vi "experiment control.vi"() -> ()   [LabVIEW 2012] (continued)
                n2481 = Concatenate Strings("ST" ("string"), w5561, "MS" ("string")) -> (w5558:string)
                n2482 = VISA Write(VISA resource name=w5564, write buffer=w5558, error in (no error)=w5565) -> (VISA resource name out=w5563:refnum<visa-resource-name>, error out=w5566:errorcluster)  [unwired: 1 out]
                n2483 = Bundle By Name(cluster=w5568, "GPIB Port"=w5563) -> (w5567:T27)
                n2484 = local write "HP8341B"(w5567) -> ()
              }
            }
          }
          frame "Microwave: Set Sweep" {
            # "Use this as a template for any command that you might want to profile."
            n2485 = local read "HP8341B"() -> (w5573:T27)
            n2486 = Unbundle By Name(w5573) -> ("detected"=w5570:bool, "Chirp"=w5571:bool)
            n2487 = And(x=w5570, y=w5571) -> (x .and. y?=w5572:bool)
            n2488 = case shown="True" w5572 {
              tunnel: w5573 -> [_ w5594]
              tunnel: [w5577 w5592] -> w5574
              tunnel: w5575 -> [w5577 w5591]
              frame False {
              }
              frame True {
                n2489 = Unbundle By Name(w5594) -> ("GPIB Port"=w5590:refnum<visa-resource-name>, "Set frequency"=w5588:dbl, "stop frequency"=w5584:dbl)
                n2490 = Number To Fractional String(number=w5588) -> (F-format string=w5587:string)  [unwired: 3 in]
                n2491 = Number To Fractional String(number=w5584) -> (F-format string=w5581:string)  [unwired: 3 in]
                n2492 = Concatenate Strings("FA" ("string"), w5587, "MZ" ("string"), "FB" ("string"), w5581, "MZ" ("string"), "S1" ("string"), "T3" ("string")) -> (w5585:string)
                n2493 = VISA Write(VISA resource name=w5590, write buffer=w5585, error in (no error)=w5591) -> (VISA resource name out=w5589:refnum<visa-resource-name>, error out=w5592:errorcluster)  [unwired: 1 out]
                n2494 = Bundle By Name(cluster=w5594, "GPIB Port"=w5589) -> (w5593:T27)
                n2495 = local write "HP8341B"(w5593) -> ()
              }
            }
          }
        }
      }
      frame #2 {
        n2496 = Unbundle By Name(w5599) -> ("Command Names"=w5603:string[])
        n2497 = Tick Count (ms)() -> (millisecond timer value=w5604:u32)
        n2498 = Search 1D Array(1D array=w5603, element=w5600) -> (index of element=w5596:i32)  [unwired: 1 in]
        n2499 = Subtract(x=w5604, y=w5598) -> (x-y=w5602:u32)
        n2500 = local read "debug timing"() -> (w5597:cluster{"command":string, "time":dbl}[])
        n2501 = Bundle("Current State"=w5600, w5602) -> (w5595:cluster{"Current State":string, u32})  [unwired: 1 in]
        n2502 = Greater Or Equal To 0?(x=w5596) -> (x >= 0?=w5601:bool)
        n2503 = case shown="False" w5601 {
          tunnel: w5597 -> [_ w5608]
          tunnel: w5596 -> [_ w5607]
          tunnel: w5595 -> [_ w5605]
          frame False {
          }
          frame True {
            n2504 = Replace Array Subset(array=w5608, new element=w5605, index=w5607) -> (→"debug timing":cluster{"command":string, "time":dbl}[])
          }
        }
      }
    }
  }
  n2505 = disable-structure shown="Enabled" {
    disable-tunnel: w1 -> [w5609 _]
    frame Enabled {
      n2506 = while "User Interface Loop" {
        tunnel: w5609 -> [w5613]
        stop <- w5610 stop-if-true
        n2507 = event shown="[13] \"save\": Value Change" {
          selector: _ -> [_ _ _ _ _ _ _ _ _ _ _ _ _ _ _ _ _ _ _ _ _ _ _ _ _ _ _ _ _ _ _ _ _ _ _ _ _ _ _ _ _ _ _ _ _ _ _ _ _ _ _ _ _ _ _ _ _ _ _ _ _ _ _]
          dyn-events: _ -> [_ _ _ _ _ _ _ _ _ _ _ _ _ _ _ _ _ _ _ _ _ _ _ _ _ _ _ _ _ _ _ _ _ _ _ _ _ _ _ _ _ _ _ _ _ _ _ _ _ _ _ _ _ _ _ _ _ _ _ _ _ _ _]
          timeout: 1000 -> [_ _ _ _ _ _ _ _ _ _ _ _ _ _ _ _ _ _ _ _ _ _ _ _ _ _ _ _ _ _ _ _ _ _ _ _ _ _ _ _ _ _ _ _ _ _ _ _ _ _ _ _ _ _ _ _ _ _ _ _ _ _ _]
          tunnel: w5613 -> [w5617 w5631 w5660 w5670 w5672 w5794 w5803 w5805 w5809 w5812 w5815 w5818 w5821 w5824 w5830 w5833 w5836 w5839 w5842 w5848 w5854 w5861 w5864 w5893 w5911 w5933 w5940 w5970 w5973 w5976 w5979 w5982 w5986 w5993 w6004 w6010 w6013 w6019 w6022 w6025 w6028 w6031 w6037 w6040 w6043 w6046 w6049 w6052 w6055 w6058 w6061 w6070 w6079 w6088 w6097 w6102 w6108 w6113 w6116 w6119 w6122 w6123 w6152]
          tunnel: [w5617 w5631 w5660 w5670 w5672 w5794 w5802 w5804 w5808 w5811 w5814 w5817 w5820 w5823 w5829 w5832 w5835 w5838 w5841 w5848 w5853 w5860 w5863 w5893 w5910 w5933 w5940 w5969 w5972 w5975 w5978 w5981 w5985 w5992 w6003 w6009 w6012 w6018 w6021 w6024 w6027 w6030 w6036 w6039 w6042 w6045 w6048 w6051 w6054 w6057 w6060 w6069 w6078 w6087 w6096 w6101 w6107 w6112 w6115 w6118 w6121 w6123 w6151] -> w5611
          event Timeout {
            n2508 = event-data() -> ()  [unwired: 1 in, 2 out]
            n2509 = Get Date/Time String(want seconds? (F)=TRUE) -> (date string=w5623:string, time string=w5624:string)  [unwired: 2 in]
            n2510 = Get Queue Status(queue=w5617, return elements? (F)=TRUE) -> (error out=w5616:errorcluster, elements=w5621:string[])  [unwired: 1 in, 6 out]
            n2511 = local write "Time"(w5624) -> ()
            n2512 = local write "Date"(w5623) -> ()
            n2513 = Search 1D Array(1D array=w5621, element="Idle") -> (index of element=w5619:i32)  [unwired: 1 in]
            n2514 = Less Than 0?(x=w5619) -> (x < 0?=w5618:bool)
            n2515 = case shown="True" w5618 {
              tunnel: w5617 -> [_ w5630]
              tunnel: w5616 -> [w5626 w5628]
              tunnel: [w5626 w5627] -> w5615
              frame False {
              }
              frame True {
                n2516 = Enqueue Element(queue=w5630, element="Idle", error in (no error)=w5628) -> (error out=w5627:errorcluster)  [unwired: 1 in, 2 out]
              }
            }
            n2517 = call <vilib>:"Clear Errors.vi"("error in (no error)"=w5615) -> ()  [unwired: 6 in, 1 out]
          }
          event Menu Selection (User) {
            n2518 = event-data() -> ("ItemTag"=w5632:string)  [unwired: 1 in]
            n2519 = case shown="\"Save\"" w5632 {
              tunnel: w5631 -> [_ w5634 w5636 w5638 w5645 w5654 w5656]
              frame "", Default {
              }
              frame "Save" {
                n2520 = Enqueue Element At Opposite End(queue=w5634, element="uBinary: Save >> Prompt") -> ()  [unwired: 2 in, 3 out]
              }
              frame "Load" {
                n2521 = Enqueue Element At Opposite End(queue=w5636, element="uBinary: Load") -> ()  [unwired: 2 in, 3 out]
              }
              frame "Abort" {
                n2522 = Enqueue Element At Opposite End(queue=w5638, element="Abort") -> ()  [unwired: 2 in, 3 out]
              }
              frame "Test" {
                w5640 = "Test" ("item tag")
                n2523 = Current VI's Menubar() -> (w5641:refnum<k9>)
                n2524 = Get Menu Item Info(7:w5640, 11:w5641) -> (0:w5642:errorcluster, 3:w5644:refnum<k9>, 4:w5643:bool)  [unwired: 1 in, 4 out]
                n2525 = Not(x=w5643) -> (.not. x?=w5639:bool)
                n2526 = Set Menu Item Info(6:w5639, 7:w5640, 8:w5642, 11:w5644) -> ()  [unwired: 3 in, 2 out]
                n2527 = case shown="True" w5639 {
                  tunnel: w5645 -> [_ w5647]
                  tunnel: w5640 -> [_ w5646]
                  frame False {
                  }
                  frame True {
                    n2528 = Enqueue Element At Opposite End(queue=w5647, element=w5646) -> ()  [unwired: 2 in, 3 out]
                  }
                }
              }
              frame "Pause" {
                w5649 = "Pause" ("item tag")
                n2529 = Current VI's Menubar() -> (w5650:refnum<k9>)
                n2530 = Get Menu Item Info(7:w5649, 11:w5650) -> (0:w5651:errorcluster, 3:w5653:refnum<k9>, 4:w5652:bool)  [unwired: 1 in, 4 out]
                n2531 = Not(x=w5652) -> (.not. x?=w5648:bool)
                n2532 = Set Menu Item Info(6:w5648, 7:w5649, 8:w5651, 11:w5653) -> ()  [unwired: 3 in, 2 out]
                n2533 = Enqueue Element At Opposite End(queue=w5654, element=w5649) -> ()  [unwired: 2 in, 3 out]
              }
              frame "Quit" {
                n2534 = Enqueue Element At Opposite End(queue=w5656, element="Macro: Exit") -> ()  [unwired: 2 in, 3 out]
              }
            }
          }
          event "Help Function Names": Double Click {
            n2535 = event-data() -> ("Row"=w5659:i32)  [unwired: 1 in]
            n2536 = property on="Help Function Names" class="LstBox (strict)"() -> ("Item Names"=w5658:string[])  [unwired: 2 in, 2 out]
            n2537 = Index Array(array=w5658, index=w5659) -> (element=w5657:string)
            n2538 = local write "stdin"(w5657) -> ()
          }
          event Shortcut Menu Activation? {
            n2539 = event-data() -> ("MenuRef"=w5663:refnum<k9>, "SubObj"=w5662:refnum<vi>)  [unwired: 1 in]
            n2540 = property class="Ctl"(reference=w5662) -> (error out=w5665:errorcluster, "Label.Text"=w5668:string)  [unwired: 1 in, 1 out]
            n2541 = Concatenate Strings("Load ", w5668, " from uBinary" ("string")) -> (w5666:string)
            n2542 = Insert Menu Items(4:w5666, 6:w5665, 8:w5666, 9:w5663) -> (0:w5664:errorcluster)  [unwired: 2 in, 2 out]
            n2543 = call <vilib>:"Clear Errors.vi"("error in (no error)"=w5664) -> ()  [unwired: 6 in, 1 out]
            n2544 = event-data("Discard?"=FALSE) -> ()  [unwired: 1 in, 1 out]
          }
          event Shortcut Menu Selection (User) {
            n2545 = event-data() -> ("ItemTag"=w5671:string)  [unwired: 1 in]
            n2546 = xnode "Match Regular Expression"("input string"=w5671, "regular expression"="Load (.+) from uBinary") -> ("offset past match"=w5675:i32, "submatch 1"=w5673:string)  [unwired: 4 in, 4 out]
            n2547 = Greater Or Equal To 0?(x=w5675) -> (x >= 0?=w5674:bool)
            n2548 = case shown="True" w5674 {
              tunnel: w5672 -> [_ w5680]
              tunnel: w5673 -> [_ w5678]
              frame False {
              }
              frame True {
                n2549 = Concatenate Strings("uBinary: Load >> " ("string"), w5678) -> (w5679:string)
                n2550 = Enqueue Element At Opposite End(queue=w5680, element=w5679) -> ()  [unwired: 2 in, 3 out]
              }
            }
          }
          event "stdin": Key Down {
            n2551 = event-data() -> ("ScanCode"=w5795:i16)  [unwired: 1 in]
            n2552 = case shown="28" w5795 {
              tunnel: w5794 -> [_ w5796]
              frame 0, Default {
              }
              frame 28 {
                # "User Presses Enter"
                n2553 = stacked-sequence {
                  tunnel: [_ w5799 _] -> w5797
                  frame #0 {
                    n2554 = property on="stdin" class="Str"("Text.Selection"=T116 {"Selection Start"=0, "Selection End"=4294967295}) -> ()  [unwired: 2 in, 2 out]
                  }
                  frame #1 {
                    n2555 = local read "stdin"() -> (w5799:string)
                  }
                  frame #2 {
                    n2556 = property on="stdin" class="Str"("Key Focus"=TRUE) -> ()  [unwired: 2 in, 2 out]
                  }
                }
                n2557 = Enqueue Element At Opposite End(queue=w5796, element=w5797) -> ()  [unwired: 2 in, 3 out]
              }
            }
          }
          event "State Hierarchy", "Machine State": Value Change {
            n2558 = event-data() -> ()  [unwired: 1 in, 5 out]
            n2559 = Enqueue Element(queue=w5803, element="Switch: Update Hierarchy") -> (queue out=w5802:refnum<queue>)  [unwired: 2 in, 2 out]
          }
          event "stop": Value Change {
            # "Exit Button Value Change (pressed) Event\n(this executes Macro: Exit to terminate the VI)"
            n2560 = event-data() -> ()  [unwired: 1 in, 5 out]
            n2561 = Enqueue Element At Opposite End(queue=w5805, element="Macro: Exit") -> (queue out=w5804:refnum<queue>)  [unwired: 2 in, 2 out]
          }
          event "Machine State.Brot": Value Change {
            n2562 = event-data() -> ()  [unwired: 1 in, 5 out]
            n2563 = Enqueue Element At Opposite End(queue=w5809, element="Switch: Set >> Brot" ("State(s) in Front (\"\")")) -> (queue out=w5808:refnum<queue>)  [unwired: 2 in, 2 out]
          }
          event "Machine State.Doublet": Value Change {
            n2564 = event-data() -> ()  [unwired: 1 in, 5 out]
            n2565 = Enqueue Element At Opposite End(queue=w5812, element="Switch: Set >> Doublet" ("State(s) in Front (\"\")")) -> (queue out=w5811:refnum<queue>)  [unwired: 2 in, 2 out]
          }
          event "Machine State.Rotation": Value Change {
            n2566 = event-data() -> ()  [unwired: 1 in, 5 out]
            n2567 = Enqueue Element At Opposite End(queue=w5815, element="Switch: Set >> Rotation" ("State(s) in Front (\"\")")) -> (queue out=w5814:refnum<queue>)  [unwired: 2 in, 2 out]
          }
          event "Machine State.Depletion phase": Value Change {
            n2568 = event-data() -> ()  [unwired: 1 in, 5 out]
            n2569 = Enqueue Element At Opposite End(queue=w5818, element="Switch: Set >> Depletion phase" ("State(s) in Front (\"\")")) -> (queue out=w5817:refnum<queue>)  [unwired: 2 in, 2 out]
          }
          event "Machine State.Depletion pol": Value Change {
            n2570 = event-data() -> ()  [unwired: 1 in, 5 out]
            n2571 = Enqueue Element At Opposite End(queue=w5821, element="Switch: Set >> Readout" ("State(s) in Front (\"\")")) -> (queue out=w5820:refnum<queue>)  [unwired: 2 in, 2 out]
          }
          event "save": Value Change {
            n2572 = event-data() -> ()  [unwired: 1 in, 5 out]
            n2573 = Enqueue Element At Opposite End(queue=w5824, element="uBinary: Save >> Prompt" ("State(s) in Front (\"\")")) -> (queue out=w5823:refnum<queue>)  [unwired: 2 in, 2 out]
          }
          event "TiSapph.setpoint": Value Change {
            n2574 = event-data() -> ()  [unwired: 1 in, 5 out]
            n2575 = local read "TiSapph"() -> (w5825:T18)
            n2576 = Unbundle By Name(w5825) -> ("setpoint"=w5827:dbl)
            n2577 = Bundle By Name(cluster=w5825, "scan start"=w5827) -> (w5826:T18)
            n2578 = Enqueue Element At Opposite End(queue=w5830, element="Laser: Start Scan >> TiSapph" ("State(s) in Front (\"\")")) -> (queue out=w5829:refnum<queue>)  [unwired: 2 in, 2 out]
            n2579 = local write "TiSapph"(w5826) -> ()
          }
          event "load": Value Change {
            n2580 = event-data() -> ()  [unwired: 1 in, 5 out]
            n2581 = Enqueue Element At Opposite End(queue=w5833, element="uBinary: Load" ("State(s) in Front (\"\")")) -> (queue out=w5832:refnum<queue>)  [unwired: 2 in, 2 out]
          }
          event "Trap DDS.channels": Value Change {
            n2582 = event-data() -> ()  [unwired: 1 in, 5 out]
            n2583 = Enqueue Element At Opposite End(queue=w5836, element="Trap DDS: Upload" ("State(s) in Front (\"\")")) -> (queue out=w5835:refnum<queue>)  [unwired: 2 in, 2 out]
          }
          event "DIO64 Override": Value Change {
            n2584 = event-data() -> ()  [unwired: 1 in, 5 out]
            n2585 = Enqueue Element At Opposite End(queue=w5839, element="DIO64: Override" ("State(s) in Front (\"\")")) -> (queue out=w5838:refnum<queue>)  [unwired: 2 in, 2 out]
          }
          event "DIO64 Tasks": Value Change {
            n2586 = event-data() -> ()  [unwired: 1 in, 5 out]
            n2587 = Enqueue Element At Opposite End(queue=w5842, element="UI: DIO64 Update Control" ("State(s) in Front (\"\")")) -> (queue out=w5841:refnum<queue>)  [unwired: 2 in, 2 out]
          }
          event "Trap DDS.ioupdate": Value Change {
            n2588 = event-data() -> ()  [unwired: 1 in, 5 out]
            n2589 = local read "Trap DDS"() -> (w5845:T26)
            n2590 = Unbundle By Name(w5845) -> ("usb 1"=w5843:refnum<visa-resource-name>, "usb 2"=w5844:refnum<visa-resource-name>)
            n2591 = Bundle By Name(cluster=w5845, "ioupdate"=FALSE) -> (w5847:T26)
            n2592 = call "DDS9959 IO Update.vi"("VISA resource name"=w5843) -> ()  [unwired: 5 in, 2 out]
            n2593 = call "DDS9959 IO Update.vi"("VISA resource name"=w5844) -> ()  [unwired: 5 in, 2 out]
            n2594 = local write "Trap DDS"(w5847) -> ()
          }
          event "Abort": Value Change {
            n2595 = event-data() -> ()  [unwired: 1 in, 5 out]
            n2596 = Enqueue Element At Opposite End(queue=w5854, element="Abort") -> (queue out=w5853:refnum<queue>)  [unwired: 2 in, 2 out]
            n2597 = call <vilib>:"Create Rendezvous.vi"("return existing (F)"=TRUE, "name (unnamed)"="sync") -> ("error out"=w5852:errorcluster, "rendezvous"=w5850:T56)  [unwired: 3 in, 1 out]
            n2598 = case shown="No Error" w5852 {
              tunnel: w5850 -> [w5857 _]
              tunnel: w5852 -> [w5856 w5858]
              frame No Error {
                n2599 = call <vilib>:"Wait at Rendezvous.vi"("error in (no error)"=w5856, "rendezvous"=w5857) -> ()  [unwired: 3 in, 3 out]
              }
              frame Error {
                n2600 = call <vilib>:"Clear Errors.vi"("error in (no error)"=w5858) -> ()  [unwired: 6 in, 1 out]
              }
            }
          }
          event "Test": Value Change {
            n2601 = event-data() -> ()  [unwired: 1 in, 5 out]
            n2602 = Enqueue Element At Opposite End(queue=w5861, element="Test") -> (queue out=w5860:refnum<queue>)  [unwired: 2 in, 2 out]
          }
          event "Measure": Value Change {
            n2603 = event-data() -> ()  [unwired: 1 in, 5 out]
            n2604 = local read "Measure Commands"() -> (w5866:string)
            n2605 = while {
              shift-right: [w5875] -> _
              shift-left: w5866 -> [w5877]
              tunnel: [w5874] -> w5862 mode=indexing
              stop <- w5872 stop-if-true
              n2606 = Match Pattern(string=w5877, regular expression="[\\n\\r]+") -> (before substring=w5874:string, after substring=w5875:string, offset past match=w5873:i32)  [unwired: 1 in, 1 out]
              n2607 = Less Than 0?(x=w5873) -> (x < 0?=w5872:bool)
            }
            n2608 = for {
              tunnel: [w5871] -> w5863
              tunnel: w5864 -> [w5870]
              shift-right: [w5868] -> w5865
              shift-left: _ -> [w5869]
              tunnel: w5862 -> [w5867] mode=indexing
              n2609 = Enqueue Element(queue=w5870, element=w5867, error in (no error)=w5869) -> (queue out=w5871:refnum<queue>, error out=w5868:errorcluster)  [unwired: 1 in, 1 out]
            }
            n2610 = call <vilib>:"Clear Errors.vi"("error in (no error)"=w5865) -> ()  [unwired: 6 in, 1 out]
          }
          event "DIO64 Tasks": Mouse Down {
            n2611 = event-data() -> ("Button"=w5878:u16, "Coords.Vertical"=w5879:i32)  [unwired: 1 in]
            n2612 = property on="DIO64 Tasks" class="Arr (strict)"() -> ("Top"=w5881:i32, "Height"=w5880:u32)  [unwired: 2 in, 2 out]
            n2613 = formula code="Y = (X-T-23)/(H-27);"("H"=w5880, "T"=w5881, "X"=w5879) -> ("Y"=w5885:dbl)
            n2614 = property on="DIO64 Tasks" class="Arr (strict)"() -> ("Number of Rows"=w5882:u32, "Index Values"=w5889:u32[])  [unwired: 2 in, 2 out]
            n2615 = In Range and Coerce(upper limit=1.0, x=w5885, lower limit=0.0) -> (coerced(x)=w5886:dbl)  [unwired: 1 out]
            n2616 = Multiply(x=w5886, y=w5882) -> (x*y=w5887:dbl)
            n2617 = Index Array(array=w5889) -> (element=w5890:u32)  [unwired: 1 in]
            n2618 = Round Toward -Infinity(1:w5887) -> (0:w5888:dbl)
            n2619 = Add(x=w5888, y=w5890) -> (x+y=w5891:dbl)
            n2620 = To Long Integer(number=w5891) -> (32bit integer=w5892:i32)
            n2621 = case shown="1" w5878 {
              selector: w5878 -> [_ _ w5898]
              tunnel: w5892 -> [_ w5894 w5897]
              frame 0, Default {
              }
              frame 3 {
                n2622 = local read "DIO64 Tasks"() -> (w5896:T4)
                n2623 = Delete From Array(array=w5896, index=w5894) -> (array with subset deleted=w5895:T4)  [unwired: 1 in, 1 out]
                n2624 = local write "DIO64 Tasks"(w5895) -> ()
              }
              frame 1 {
                n2625 = disable-structure shown="Disabled" {
                  disable-tunnel: w5898 -> [w5901 _]
                  disable-tunnel: w5897 -> [w5899 _]
                  frame Disabled {
                    n2626 = Bundle(w5899, "Button"=w5901) -> (w5900:cluster{i32, "Button":u16})  [unwired: 1 in]
                    n2627 = Bundle("dio64_task_drag", w5900) -> (w5903:cluster{string, cluster{i32, "Button":u16}})  [unwired: 1 in]
                    n2628 = Build Array(w5903) -> (w5902:cluster{string, cluster{i32, "Button":u16}}[])
                    n2629 = invoke on="DIO64 Tasks" class="Arr (strict)" method="Start Drag"("Data"=w5902, "AllowsMove"=enum32{"copy or move", "copy only", "move only"}."move only" ("Drag Mode")) -> ()  [unwired: 3 in, 5 out]
                  }
                  frame Enabled {
                  }
                }
              }
            }
          }
          event "pause:skip": Value Change {
            n2630 = event-data() -> ()  [unwired: 1 in, 1 out]
            n2631 = Select(t="Pause" ("element"), s="pause:skip", f="Unpause" ("element")) -> (s? t:f=w5907:string)
            n2632 = Enqueue Element(queue=w5911, element=w5907) -> (queue out=w5910:refnum<queue>)  [unwired: 2 in, 2 out]
          }
          event "DIO64": Drop {
            n2633 = event-data() -> ("Coords.Vertical"=w5912:i32)  [unwired: 1 in]
            n2634 = property on="DIO64" class="Arr (strict)"() -> ("Top"=w5914:i32, "Height"=w5913:u32)  [unwired: 2 in, 2 out]
            n2635 = formula code="Y = (X-T-23)/(H-27);"("H"=w5913, "T"=w5914, "X"=w5912) -> ("Y"=w5918:dbl)
            n2636 = property on="DIO64" class="Arr (strict)"() -> ("Number of Rows"=w5915:u32, "Index Values"=w5922:u32[])  [unwired: 2 in, 2 out]
            n2637 = Bundle("32bit integer"=0, "32bit integer"=u16 0) -> (w5927:T117)  [unwired: 1 in]
            n2638 = In Range and Coerce(upper limit=1.0, x=w5918, lower limit=0.0) -> (coerced(x)=w5919:dbl)  [unwired: 1 out]
            n2639 = Multiply(x=w5919, y=w5915) -> (x*y=w5920:dbl)
            n2640 = Index Array(array=w5922) -> (element=w5923:u32)  [unwired: 1 in]
            n2641 = Get Drag Drop Data(8:w5927, 9:"dio64_row_drag" ("data name")) -> (3:w5930:T117)  [unwired: 1 in, 1 out]
            n2642 = Round Toward -Infinity(1:w5920) -> (0:w5921:dbl)
            n2643 = Add(x=w5921, y=w5923) -> (x+y=w5924:dbl)
            n2644 = Unbundle(w5930) -> ("32bit integer"=w5932:i32, "32bit integer"=w5931:u16)
            n2645 = To Long Integer(number=w5924) -> (32bit integer=w5925:i32)
            n2646 = case shown="2" w5931 {
              tunnel: w5925 -> [_ w5935]
              tunnel: w5932 -> [_ w5934]
              frame 0, Default {
              }
              frame 2 {
                n2647 = local read "DIO64"() -> (w5937:T3)
                n2648 = Delete From Array(array=w5937, index=w5934) -> (deleted portion=w5938:T93, array with subset deleted=w5939:T3)  [unwired: 1 in]
                n2649 = Insert Into Array(array=w5939, index=w5935, new element=w5938) -> (w5936:T3)
                n2650 = local write "DIO64"(w5936) -> ()
              }
            }
            n2651 = event-data() -> ()  [unwired: 2 in, 1 out]
          }
          event "DIO64 Tasks": Drop {
            n2652 = event-data() -> ("Coords.Vertical"=w5941:i32)  [unwired: 1 in]
            n2653 = property on="DIO64 Tasks" class="Arr (strict)"() -> ("Top"=w5943:i32, "Height"=w5942:u32)  [unwired: 2 in, 2 out]
            n2654 = formula code="Y = (X-T-23)/(H-27);"("H"=w5942, "T"=w5943, "X"=w5941) -> ("Y"=w5947:dbl)
            n2655 = property on="DIO64 Tasks" class="Arr (strict)"() -> ("Number of Rows"=w5944:u32, "Index Values"=w5951:u32[])  [unwired: 2 in, 2 out]
            n2656 = Bundle("32bit integer"=0, "32bit integer"=u16 0) -> (w5956:T117)  [unwired: 1 in]
            n2657 = In Range and Coerce(upper limit=1.0, x=w5947, lower limit=0.0) -> (coerced(x)=w5948:dbl)  [unwired: 1 out]
            n2658 = Multiply(x=w5948, y=w5944) -> (x*y=w5949:dbl)
            n2659 = Index Array(array=w5951) -> (element=w5952:u32)  [unwired: 1 in]
            n2660 = Get Drag Drop Data(8:w5956, 9:"dio64_task_drag" ("data name")) -> (3:w5959:T117)  [unwired: 1 in, 1 out]
            n2661 = Round Toward -Infinity(1:w5949) -> (0:w5950:dbl)
            n2662 = Add(x=w5950, y=w5952) -> (x+y=w5953:dbl)
            n2663 = Unbundle(w5959) -> ("32bit integer"=w5961:i32, "32bit integer"=w5960:u16)
            n2664 = To Long Integer(number=w5953) -> (32bit integer=w5954:i32)
            n2665 = case shown="2" w5960 {
              tunnel: w5954 -> [_ w5963]
              tunnel: w5961 -> [_ w5962]
              frame 0, Default {
              }
              frame 2 {
                n2666 = local read "DIO64 Tasks"() -> (w5965:T4)
                n2667 = Delete From Array(array=w5965, index=w5962) -> (deleted portion=w5966:T118, array with subset deleted=w5967:T4)  [unwired: 1 in]
                n2668 = Insert Into Array(array=w5967, index=w5963, new element=w5966) -> (w5964:T4)
                n2669 = local write "DIO64 Tasks"(w5964) -> ()
              }
            }
            n2670 = event-data() -> ()  [unwired: 2 in, 1 out]
          }
          event "DAC Upload": Value Change {
            n2671 = event-data() -> ()  [unwired: 1 in, 5 out]
            n2672 = Enqueue Element At Opposite End(queue=w5970, element="DAC: Upload2") -> (queue out=w5969:refnum<queue>)  [unwired: 2 in, 2 out]
          }
          event "DIO64": Value Change {
            n2673 = event-data() -> ()  [unwired: 1 in, 5 out]
            n2674 = Enqueue Element At Opposite End(queue=w5973, element="DIO64: Update Graph") -> (queue out=w5972:refnum<queue>)  [unwired: 2 in, 2 out]
          }
          event "Channel Labels": Value Change {
            n2675 = event-data() -> ()  [unwired: 1 in, 5 out]
            n2676 = Enqueue Element At Opposite End(queue=w5976, element="UI: DIO64 Change Labels") -> (queue out=w5975:refnum<queue>)  [unwired: 2 in, 2 out]
          }
          event "Chop Labels": Value Change {
            n2677 = event-data() -> ()  [unwired: 1 in, 5 out]
            n2678 = Enqueue Element At Opposite End(queue=w5979, element="UI: Chop Labels") -> (queue out=w5978:refnum<queue>)  [unwired: 2 in, 2 out]
          }
          event "Wavemaster.Units": Value Change {
            n2679 = event-data() -> ()  [unwired: 1 in, 5 out]
            n2680 = Enqueue Element At Opposite End(queue=w5982, element="Wavemeter: Set Units") -> (queue out=w5981:refnum<queue>)  [unwired: 2 in, 2 out]
          }
          event "Abby Reset": Value Change {
            n2681 = event-data() -> ()  [unwired: 1 in, 5 out]
            n2682 = Reverse 1D Array(array=string[] ["USB DAQ: Digital Write >> 2,1", "USB DAQ: Digital Write >> 2,0", "USB DAQ: Digital Write >> 1,1", "USB DAQ: Digital Write >> 1,0", "Wait >> 10", ""]) -> (reversed array=w5983:string[])
            n2683 = for {
              shift-right: [w5988] -> w5985
              shift-left: w5986 -> [w5989]
              tunnel: w5983 -> [w5987] mode=indexing
              n2684 = Enqueue Element At Opposite End(queue=w5989, element=w5987) -> (queue out=w5988:refnum<queue>)  [unwired: 2 in, 2 out]
            }
          }
          event "Abby Disable": Value Change {
            n2685 = event-data() -> ()  [unwired: 1 in, 5 out]
            n2686 = Reverse 1D Array(array=string[] ["USB DAQ: Digital Write >> 2,1", "USB DAQ: Digital Write >> 2,0", "Wait >> 10"]) -> (reversed array=w5990:string[])
            n2687 = for {
              shift-right: [w5995] -> w5992
              shift-left: w5993 -> [w5996]
              tunnel: w5990 -> [w5994] mode=indexing
              n2688 = Enqueue Element At Opposite End(queue=w5996, element=w5994) -> (queue out=w5995:refnum<queue>)  [unwired: 2 in, 2 out]
            }
          }
          event "Bertha Flip": Value Change {
            n2689 = event-data() -> ("NewVal"=w5997:bool)  [unwired: 1 in, 4 out]
            n2690 = Boolean To (0,1)(Boolean=w5997) -> (0, 1=w6002:i16)
            n2691 = Number To Decimal String(number=w6002) -> (decimal integer string=w6000:string)  [unwired: 1 in]
            n2692 = Concatenate Strings("USB DAQ: Digital Write >> 3,", w6000) -> (w5999:string)
            n2693 = Build Array(w5999) -> (w5998:string[])
            n2694 = for {
              shift-right: [w6006] -> w6003
              shift-left: w6004 -> [w6007]
              tunnel: w5998 -> [w6005] mode=indexing
              n2695 = Enqueue Element At Opposite End(queue=w6007, element=w6005) -> (queue out=w6006:refnum<queue>)  [unwired: 2 in, 2 out]
            }
          }
          event "Clear IMG MCP": Value Change {
            n2696 = event-data() -> ()  [unwired: 1 in, 5 out]
            n2697 = Enqueue Element At Opposite End(queue=w6010, element="IMG MCP: Clear") -> (queue out=w6009:refnum<queue>)  [unwired: 2 in, 2 out]
          }
          event "USB DAQ.Digital Out": Value Change {
            n2698 = event-data() -> ()  [unwired: 1 in, 5 out]
            n2699 = Enqueue Element At Opposite End(queue=w6013, element="USB DAQ: Digital Write") -> (queue out=w6012:refnum<queue>)  [unwired: 2 in, 2 out]
          }
          event "Trap Agilent.Upload": Value Change {
            n2700 = event-data() -> ()  [unwired: 1 in, 5 out]
            n2701 = local read "Trap Agilent"() -> (w6015:T13)
            n2702 = Bundle By Name(cluster=w6015, "Upload"=FALSE) -> (w6014:T13)
            n2703 = local write "Trap Agilent"(w6014) -> ()
            n2704 = Enqueue Element At Opposite End(queue=w6019, element="Trap Agilent: Set") -> (queue out=w6018:refnum<queue>)  [unwired: 2 in, 2 out]
          }
          event "Trap Agilent.Output": Value Change {
            n2705 = event-data() -> ()  [unwired: 1 in, 5 out]
            n2706 = Enqueue Element At Opposite End(queue=w6022, element="Trap Agilent: Output") -> (queue out=w6021:refnum<queue>)  [unwired: 2 in, 2 out]
          }
          event "Chillax.Output": Value Change {
            n2707 = event-data() -> ()  [unwired: 1 in, 5 out]
            n2708 = Enqueue Element At Opposite End(queue=w6025, element="Chillax: Output") -> (queue out=w6024:refnum<queue>)  [unwired: 2 in, 2 out]
          }
          event "Chillax.Chillax Voltage": Value Change {
            n2709 = event-data() -> ()  [unwired: 1 in, 5 out]
            n2710 = Enqueue Element At Opposite End(queue=w6028, element="Chillax: Set Voltage") -> (queue out=w6027:refnum<queue>)  [unwired: 2 in, 2 out]
          }
          event "DAC Schedule": Value Change {
            n2711 = event-data() -> ()  [unwired: 1 in, 5 out]
            n2712 = Enqueue Element At Opposite End(queue=w6031, element="DAC: View") -> (queue out=w6030:refnum<queue>)  [unwired: 2 in, 2 out]
          }
          event "Depletion Agilent.Channels", "Depletion Agilent.Upload": Value Change {
            n2713 = event-data() -> ()  [unwired: 1 in, 5 out]
            n2714 = local read "Depletion Agilent"() -> (w6033:T14)
            n2715 = Bundle By Name(cluster=w6033, "Upload"=FALSE) -> (w6032:T14)
            n2716 = local write "Depletion Agilent"(w6032) -> ()
            n2717 = Enqueue Element At Opposite End(queue=w6037, element="Depletion Agilent: Set") -> (queue out=w6036:refnum<queue>)  [unwired: 2 in, 2 out]
          }
          event "Depletion Agilent.Output": Value Change {
            n2718 = event-data() -> ()  [unwired: 1 in, 5 out]
            n2719 = Enqueue Element At Opposite End(queue=w6040, element="Depletion Agilent: Output") -> (queue out=w6039:refnum<queue>)  [unwired: 2 in, 2 out]
          }
          event "USB DAQ.Analog Out": Value Change {
            n2720 = event-data() -> ()  [unwired: 1 in, 5 out]
            n2721 = Enqueue Element At Opposite End(queue=w6043, element="USB DAQ: Analog Write") -> (queue out=w6042:refnum<queue>)  [unwired: 2 in, 2 out]
          }
          event "Coils.Current Toggle": Value Change {
            n2722 = event-data() -> ()  [unwired: 1 in, 5 out]
            n2723 = Enqueue Element At Opposite End(queue=w6046, element="Coils: Set") -> (queue out=w6045:refnum<queue>)  [unwired: 2 in, 2 out]
          }
          event "Coils.Magnetometer Shim": Value Change {
            n2724 = event-data() -> ()  [unwired: 1 in, 5 out]
            n2725 = Enqueue Element At Opposite End(queue=w6049, element="Coils: Set") -> (queue out=w6048:refnum<queue>)  [unwired: 2 in, 2 out]
          }
          event "Coils.Ion Shim": Value Change {
            n2726 = event-data() -> ()  [unwired: 1 in, 5 out]
            n2727 = Enqueue Element At Opposite End(queue=w6052, element="Coils: Set") -> (queue out=w6051:refnum<queue>)  [unwired: 2 in, 2 out]
          }
          event "Coils.Bias": Value Change {
            n2728 = event-data() -> ()  [unwired: 1 in, 5 out]
            n2729 = Enqueue Element At Opposite End(queue=w6055, element="Coils: Set") -> (queue out=w6054:refnum<queue>)  [unwired: 2 in, 2 out]
          }
          event "Coils.Total": Value Change {
            n2730 = event-data() -> ()  [unwired: 1 in, 5 out]
            n2731 = Enqueue Element At Opposite End(queue=w6058, element="Coils: Set") -> (queue out=w6057:refnum<queue>)  [unwired: 2 in, 2 out]
          }
          event "DDS.clock": Value Change {
            n2732 = event-data() -> ()  [unwired: 1 in, 5 out]
            n2733 = Enqueue Element At Opposite End(queue=w6061, element="DDS: Set Clock") -> (queue out=w6060:refnum<queue>)  [unwired: 2 in, 2 out]
          }
          event "DDS.channel 1": Value Change {
            n2734 = event-data() -> ("OldVal"=w6066:dbl, "NewVal"=w6063:dbl)  [unwired: 1 in, 3 out]
            n2735 = local read "DDS"() -> (w6067:T25)
            n2736 = Bundle By Name(cluster=w6067, "channel 1"=w6066) -> (w6068:T25)
            n2737 = local write "DDS"(w6068) -> ()
            n2738 = Number To Fractional String(number=w6063) -> (F-format string=w6064:string)  [unwired: 3 in]
            n2739 = Concatenate Strings("DDS: Goto Frequency >> 1," ("State(s) in Front (\"\")"), w6064) -> (w6062:string)
            n2740 = Enqueue Element At Opposite End(queue=w6070, element=w6062) -> (queue out=w6069:refnum<queue>)  [unwired: 2 in, 2 out]
          }
          event "DDS.channel 2": Value Change {
            n2741 = event-data() -> ("OldVal"=w6075:dbl, "NewVal"=w6072:dbl)  [unwired: 1 in, 3 out]
            n2742 = local read "DDS"() -> (w6076:T25)
            n2743 = Bundle By Name(cluster=w6076, "channel 2"=w6075) -> (w6077:T25)
            n2744 = local write "DDS"(w6077) -> ()
            n2745 = Number To Fractional String(number=w6072) -> (F-format string=w6073:string)  [unwired: 3 in]
            n2746 = Concatenate Strings("DDS: Goto Frequency >> 2," ("State(s) in Front (\"\")"), w6073) -> (w6071:string)
            n2747 = Enqueue Element At Opposite End(queue=w6079, element=w6071) -> (queue out=w6078:refnum<queue>)  [unwired: 2 in, 2 out]
          }
          event "DDS.channel 3": Value Change {
            n2748 = event-data() -> ("OldVal"=w6084:dbl, "NewVal"=w6081:dbl)  [unwired: 1 in, 3 out]
            n2749 = local read "DDS"() -> (w6085:T25)
            n2750 = Bundle By Name(cluster=w6085, "channel 3"=w6084) -> (w6086:T25)
            n2751 = local write "DDS"(w6086) -> ()
            n2752 = Number To Fractional String(number=w6081) -> (F-format string=w6082:string)  [unwired: 3 in]
            n2753 = Concatenate Strings("DDS: Goto Frequency >> 3," ("State(s) in Front (\"\")"), w6082) -> (w6080:string)
            n2754 = Enqueue Element At Opposite End(queue=w6088, element=w6080) -> (queue out=w6087:refnum<queue>)  [unwired: 2 in, 2 out]
          }
          event "DDS.channel 4": Value Change {
            n2755 = event-data() -> ("OldVal"=w6093:dbl, "NewVal"=w6090:dbl)  [unwired: 1 in, 3 out]
            n2756 = local read "DDS"() -> (w6094:T25)
            n2757 = Bundle By Name(cluster=w6094, "channel 4"=w6093) -> (w6095:T25)
            n2758 = local write "DDS"(w6095) -> ()
            n2759 = Number To Fractional String(number=w6090) -> (F-format string=w6091:string)  [unwired: 3 in]
            n2760 = Concatenate Strings("DDS: Goto Frequency >> 4," ("State(s) in Front (\"\")"), w6091) -> (w6089:string)
            n2761 = Enqueue Element At Opposite End(queue=w6097, element=w6089) -> (queue out=w6096:refnum<queue>)  [unwired: 2 in, 2 out]
          }
          event "HP8341B.frequency": Value Change {
            n2762 = event-data() -> ()  [unwired: 1 in, 5 out]
            n2763 = local read "HP8341B"() -> (w6099:T27)
            n2764 = Unbundle By Name(w6099) -> ("Chirp"=w6100:bool)
            n2765 = case shown="False" w6100 {
              tunnel: ["Microwave: Set Sweep" ("State(s) in Front (\"\")") "Microwave: Set Frequency" ("State(s) in Front (\"\")")] -> w6098
              frame True {
              }
              frame False {
              }
            }
            n2766 = Enqueue Element At Opposite End(queue=w6102, element=w6098) -> (queue out=w6101:refnum<queue>)  [unwired: 2 in, 2 out]
          }
          event "HP8341B.Chirp": Value Change {
            n2767 = event-data() -> ("NewVal"=w6106:bool)  [unwired: 1 in, 4 out]
            n2768 = case shown="True" w6106 {
              tunnel: ["Microwave: Set Sweep" ("State(s) in Front (\"\")") "Microwave: Set Frequency" ("State(s) in Front (\"\")")] -> w6105
              frame True {
              }
              frame False {
              }
            }
            n2769 = Enqueue Element At Opposite End(queue=w6108, element=w6105) -> (queue out=w6107:refnum<queue>)  [unwired: 2 in, 2 out]
          }
          event "HP8341B.rf": Value Change {
            n2770 = event-data() -> ()  [unwired: 1 in, 5 out]
            n2771 = Enqueue Element At Opposite End(queue=w6113, element="Microwave: RF" ("State(s) in Front (\"\")")) -> (queue out=w6112:refnum<queue>)  [unwired: 2 in, 2 out]
          }
          event "HP8341B.Pulse Modulate": Value Change {
            n2772 = event-data() -> ()  [unwired: 1 in, 5 out]
            n2773 = Enqueue Element At Opposite End(queue=w6116, element="Microwave: Pulse" ("State(s) in Front (\"\")")) -> (queue out=w6115:refnum<queue>)  [unwired: 2 in, 2 out]
          }
          event "HP8341B.power": Value Change {
            n2774 = event-data() -> ()  [unwired: 1 in, 5 out]
            n2775 = Enqueue Element At Opposite End(queue=w6119, element="Microwave: Set Power" ("State(s) in Front (\"\")")) -> (queue out=w6118:refnum<queue>)  [unwired: 2 in, 2 out]
          }
          event "HP8341B.stop frequency": Value Change {
            n2776 = event-data() -> ()  [unwired: 1 in, 5 out]
            n2777 = Enqueue Element At Opposite End(queue=w6122, element="Microwave: Set Sweep" ("State(s) in Front (\"\")")) -> (queue out=w6121:refnum<queue>)  [unwired: 2 in, 2 out]
          }
          event "DIO64": Mouse Down {
            n2778 = event-data() -> ("Button"=w6125:u16, "Coords.Vertical"=w6124:i32)  [unwired: 1 in]
            n2779 = property on="DIO64" class="Arr (strict)"() -> ("Top"=w6137:i32, "Height"=w6138:u32)  [unwired: 2 in, 2 out]
            n2780 = formula code="Y = (X-T-23)/(H-27);"("H"=w6138, "T"=w6137, "X"=w6124) -> ("Y"=w6133:dbl)
            n2781 = property on="DIO64" class="Arr (strict)"() -> ("Number of Rows"=w6136:u32, "Index Values"=w6129:u32[])  [unwired: 2 in, 2 out]
            n2782 = In Range and Coerce(upper limit=1.0, x=w6133, lower limit=0.0) -> (coerced(x)=w6132:dbl)  [unwired: 1 out]
            n2783 = Multiply(x=w6132, y=w6136) -> (x*y=w6131:dbl)
            n2784 = Index Array(array=w6129) -> (element=w6128:u32)  [unwired: 1 in]
            n2785 = Round Toward -Infinity(1:w6131) -> (0:w6130:dbl)
            n2786 = Add(x=w6130, y=w6128) -> (x+y=w6127:dbl)
            n2787 = To Long Integer(number=w6127) -> (32bit integer=w6126:i32)
            n2788 = case shown="1" w6125 {
              selector: w6125 -> [_ _ w6143]
              tunnel: w6126 -> [_ w6139 w6142]
              frame 0, Default {
              }
              frame 3 {
                n2789 = local read "DIO64"() -> (w6141:T3)
                n2790 = Delete From Array(array=w6141, index=w6139) -> (array with subset deleted=w6140:T3)  [unwired: 1 in, 1 out]
                n2791 = local write "DIO64"(w6140) -> ()
              }
              frame 1 {
                n2792 = disable-structure shown="Disabled" {
                  disable-tunnel: w6143 -> [w6146 _]
                  disable-tunnel: w6142 -> [w6144 _]
                  frame Disabled {
                    n2793 = Bundle(w6144, "Button"=w6146) -> (w6145:cluster{i32, "Button":u16})  [unwired: 1 in]
                    n2794 = Bundle("dio64_row_drag", w6145) -> (w6148:cluster{string, cluster{i32, "Button":u16}})  [unwired: 1 in]
                    n2795 = Build Array(w6148) -> (w6147:cluster{string, cluster{i32, "Button":u16}}[])
                    n2796 = invoke on="DIO64" class="Arr (strict)" method="Start Drag"("Data"=w6147, "AllowsMove"=enum32{"copy or move", "copy only", "move only"}."move only" ("Drag Mode")) -> ()  [unwired: 3 in, 5 out]
                  }
                  frame Enabled {
                  }
                }
              }
            }
          }
          event Panel Close? {
            # "Close Panel button (pressed) Event\n(this executes Macro: Exit to terminate the VI)"
            n2797 = event-data() -> ()  [unwired: 1 in, 3 out]
            n2798 = Enqueue Element(queue=w6152, element="Macro: Exit") -> (queue out=w6151:refnum<queue>)  [unwired: 2 in, 2 out]
            n2799 = event-data("Discard?"=TRUE) -> ()  [unwired: 1 in, 1 out]
          }
        }
        n2800 = Get Queue Status(queue=w5611, return elements? (F)=TRUE) -> (error out=w5610:errorcluster)  [unwired: 1 in, 7 out]
      }
    }
    frame Disabled {
    }
  }
  n2801 = disable-structure shown="Enabled" {
    disable-tunnel: w1 -> [w6155 _]
    frame Enabled {
      n2802 = while "Matlab Communication Loop" {
        tunnel: w6155 -> [w6159]
        stop <- w6164 stop-if-true
        w6163 = u16 8888  # port
        n2803 = call <vilib>:"TCP Listen.vi"("timeout ms (wait forever: -1)"=100, "port"=w6163) -> ("error out"=w6160:errorcluster, "connection ID"=w6161:refnum<k5>)  [unwired: 5 in, 3 out]
        n2804 = case shown="No Error" w6160 {
          tunnel: w6161 -> [w6173 _]
          tunnel: w6160 -> [w6172 _]
          tunnel: w6159 -> [w6170 w6386]
          tunnel: [w6169 w6386] -> w6158
          frame No Error {
            n2805 = TCP Read(connection ID=w6173, bytes to read=4, error in (no error)=w6172, 9:10000 ("timeout ms (25000)")) -> (connection ID out=w6179:refnum<k5>, data out=w6177:string, error out=w6178:errorcluster)  [unwired: 1 in]
            n2806 = Type Cast(type=u32 1 ("bytes to read"), x=w6177) -> (*(type *) &x=w6175:u32)
            n2807 = To Long Integer(number=w6175) -> (32bit integer=w6174:i32)
            n2808 = TCP Read(connection ID=w6179, bytes to read=w6174, error in (no error)=w6178) -> (connection ID out=w6167:refnum<k5>, data out=w6171:string, error out=w6168:errorcluster)  [unwired: 2 in]
            n2809 = case shown="\"sync\"" w6171 {
              selector: w6171 -> [w6182 _ _ _ _ _ _ _]
              tunnel: w6170 -> [w6186 w6197 w6209 w6218 w6232 w6277 w6321 w6366]
              tunnel: [w6186 w6197 w6209 w6218 w6232 w6277 w6321 w6366] -> w6169
              tunnel: w6168 -> [w6185 w6188 w6205 w6214 w6230 w6275 w6319 w6369]
              tunnel: [w6184 w6196 w6208 w6210 w6242 w6287 w6331 w6368] -> w6166
              tunnel: w6167 -> [w6183 w6192 w6203 w6215 w6231 w6276 w6320 w6365]
              tunnel: [w6183 w6191 w6202 w6219 w6241 w6286 w6330 w6364] -> w6165
              frame "", Default {
                n2810 = Enqueue Element(queue=w6186, element=w6182, error in (no error)=w6185) -> (error out=w6184:errorcluster)  [unwired: 1 in, 2 out]
              }
              frame "commands" {
                # "Send a list of commands that can be executed by the primary event loop to Matlab"
                n2811 = local read "debug timing"() -> (w6189:cluster{"command":string, "time":dbl}[])
                n2812 = for {
                  tunnel: w6189 -> [w6199] mode=indexing
                  tunnel: [w6198] -> w6187 mode=indexing
                  n2813 = Unbundle By Name(w6199) -> ("command"=w6198:string)
                }
                n2814 = Flatten To String(anything=w6187, error in (no error)=w6188) -> (data string=w6194:string, error out=w6193:errorcluster)  [unwired: 2 in, 1 out]
                n2815 = TCP Write(connection ID=w6192, data in=w6194, error in (no error)=w6193) -> (connection ID out=w6191:refnum<k5>, error out=w6195:errorcluster)  [unwired: 1 in, 1 out]
                n2816 = Enqueue Element(queue=w6197, element="Debug: Console >> Matlab is asking for a list of commands." ("string"), error in (no error)=w6195) -> (error out=w6196:errorcluster)  [unwired: 1 in, 2 out]
              }
              frame "documentation" {
                # "Sends an array of documentation strings grabbed from the text boxes in the main event loop that can be used by Matlab."
                n2817 = local read "documentation"() -> (w6200:string[])
